vi "cblas dzasum.vi"(5 "n":i32=-1, 7 "incx":i32=1, 11 "x":cdb[](array[numeric])) -> (0 "error":i32, 3 "dzasum":dbl)   [LabVIEW 2020, in "NI_AALBLAS.lvlib"]
doc: "Calculates the sum of the absolute values of elements in <B>X</B> with indexes that are multiples of <B>incX</B>. The data type you wire to the <B>X</B> input determines the polymorphic instance to use."
uses:
  NI_AALBLAS.lvlib
  <resource>/lvblas.dll
panel:
  # "double cblas_dzasum(n, *x, incx)"
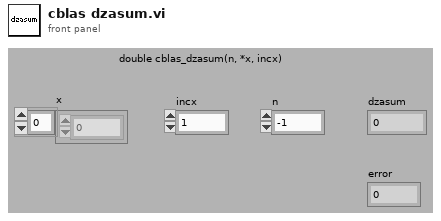
[diagram p1: front panel]
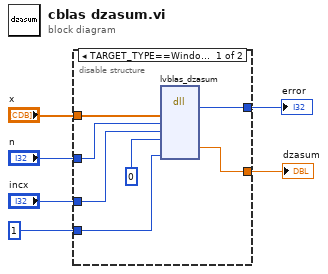
[diagram p0: block diagram]
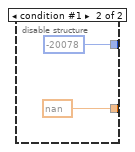
[diagram p2: hidden frame]
diagram:
  n1 = disable-structure shown="TARGET_TYPE==Windows||TARGET_TYPE==Unix||TARGET_TYPE==Mac||TARGET_TYPE==RT" {
    disable-tunnel: "x" -> [w12 _]
    disable-tunnel: "n" -> [w11 _]
    disable-tunnel: "incx" -> [w10 _]
    disable-tunnel: [w8 nan] -> w3
    disable-tunnel: [w13 -20078] -> w2
    disable-tunnel: 1 -> [w7 _]
    frame condition #0 (active) {
      n2 = dll-call lib="C:/Program Files (x86)/National Instruments/LabVIEW 2020/resource/lvblas.*" fn="lvblas_dzasum" ("LVBLAS.dll:CxBLASVectorSumH")("X"=w12, "N"=w11, "IncX"=w10, "startX"=0, "check"=w7) -> ("error"=w13:i32, "dzasum"=w8:dbl)  [unwired: 8 in, 3 out]
    }
    frame condition #1 {
    }
  }
  "dzasum" <- w3
  "error" <- w2
